vi "Date_and_Time_to_string.vi"() -> (0 "dateTime":T1(array[cluster]), 1 "Date and time (spreadsheet)":string)   [LabVIEW 2020]
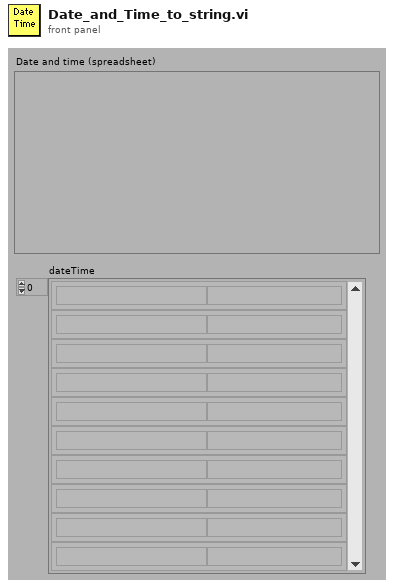
[diagram p1: front panel]
types:
  T1 = cluster{"Label.Text":string, "date/time string":string}[]
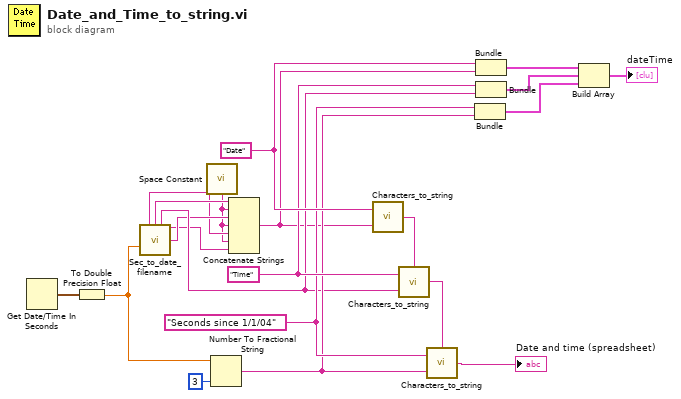
[diagram p0: block diagram]
diagram:
  w17 = "Seconds since 1/1/04"
  w18 = "Time"
  w19 = "Date"
  n1 = Get Date/Time In Seconds() -> (seconds since 1Jan1904=w20:timestamp)
  n2 = To Double Precision Float(number=w20) -> (double precision float=w9:dbl)
  n3 = call "Sec_to_date_filename.vi"("ss1904"=w9) -> ("shortMonthName"=w4:string, "shortDayName"=w6:string, "HH:MM"=w8:string, "YYYY"=w3:string, "DD"=w5:string)  [unwired: 5 in, 5 out]
  n4 = call <vilib>:"Space Constant.vi"() -> ("String"=w2:string)
  n5 = Number To Fractional String(number=w9, precision (6)=i16 3) -> (F-format string=w16:string)  [unwired: 2 out]
  n6 = Concatenate Strings(w6, w2, w5, w2, w4, w2, w3) -> (w7:string)
  n7 = call "Characters_to_string.vi"("Characters to write"=w7, "Label for characters"=w19) -> ("Output string"=w15:string)  [unwired: 1 in]
  n8 = call "Characters_to_string.vi"("stringIn"=w15, "Characters to write"=w8, "Label for characters"=w18) -> ("Output string"=w14:string)
  n9 = call "Characters_to_string.vi"("stringIn"=w14, "Characters to write"=w16, "Label for characters"=w17) -> ("Output string"=→"Date and time (spreadsheet)":string)
  n10 = Bundle(w17, w16) -> (w11:cluster{string, string})  [unwired: 1 in]
  n11 = Bundle(w19, w7) -> (w13:cluster{string, string})  [unwired: 1 in]
  n12 = Bundle(w18, "HH:MM"=w8) -> (w12:cluster{string, "HH:MM":string})  [unwired: 1 in]
  n13 = Build Array(w13, w12, w11) -> (→"dateTime":cluster{string, "HH:MM":string}[])
